vi "Map Graph XY to Panel Coordinates.vi"(1 "XY":cluster{dbl, dbl}, 2 "Graph":refnum<vi>) -> (0 "Coords":cluster{i32, i32})   [LabVIEW 2023]
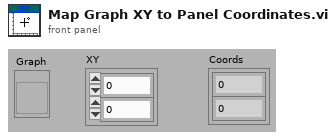
[diagram p1: front panel]
types:
  T1 = typedef "LVRectTypeDef.ctl" = cluster{"Left":i16, "Top":i16, "Right":i16, "Bottom":i16}
  T2 = typedef "LVPoint32TypeDef.ctl" = cluster{"Horizontal":i32, "Vertical":i32}
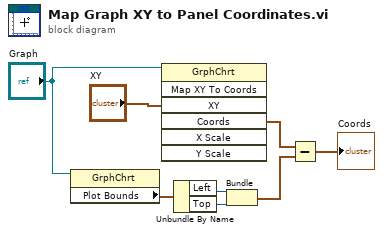
[diagram p0: block diagram]
diagram:
  n1 = property on="Property Node" class="GrphChrt"(reference="Graph") -> ("Plot Bounds"=w5:T1)  [unwired: 1 in, 2 out]
  n2 = invoke class="GrphChrt" method="Map XY To Coords"(reference="Graph", "XY"="XY") -> ("Coords"=w3:T2)  [unwired: 5 in, 6 out]
  n3 = Unbundle By Name(w5) -> ("Left"=w6:i16, "Top"=w7:i16)
  n4 = Bundle("Left"=w6, "Top"=w7) -> (w8:cluster{"Left":i16, "Top":i16})  [unwired: 1 in]
  n5 = Subtract(x=w3, y=w8) -> (x-y=→"Coords":T2)
